vi "Write VI.vi"(8 "error in (no error)":errorcluster, 10 "VI Path (.vi)":path, 11 "Snippet":T1) -> (0 "error out":errorcluster)   [LabVIEW 2022 SP3, in "VI-Snippet.lvlib"]
doc: "Writes the embedded VI to disk."
uses:
  VI-Snippet.lvlib
  Snippet.ctl
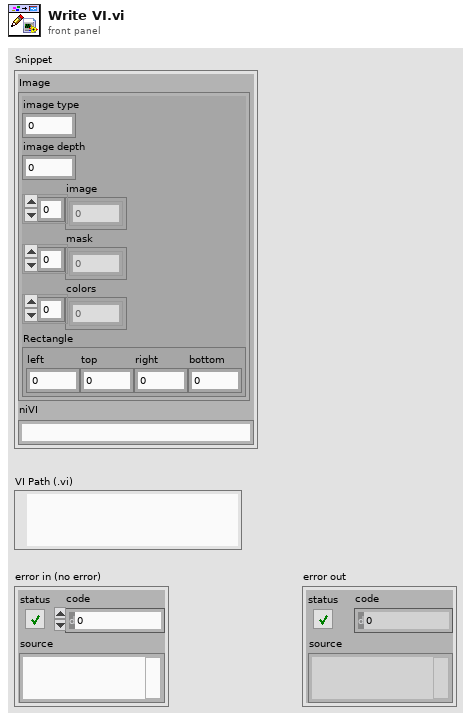
[diagram p1: front panel]
types:
  T1 = typedef "VI-Snippet.lvlib/Snippet.ctl" = cluster{"Image":cluster{"image type":i32, "image depth":i32, "image":u8[], "mask":u8[], "colors":u32[], "Rectangle":cluster{"left":i16, "top":i16, "right":i16, "bottom":i16}}, "niVI":string}
  T2 = enum16{"open", "replace", "create", "open or create", "replace or create", "replace or create with confirmation"}
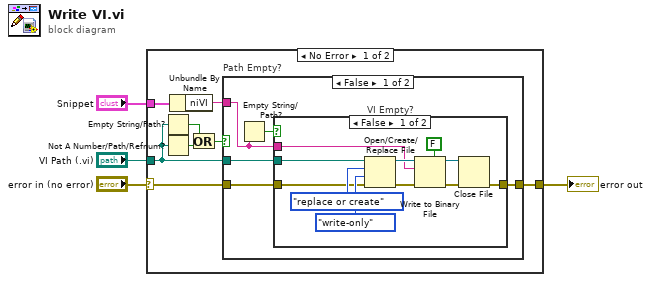
[diagram p0: block diagram]
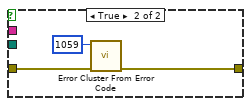
[diagram p2: hidden frame]
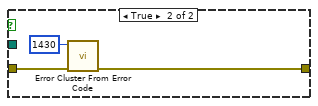
[diagram p3: hidden frame]
diagram:
  n1 = case shown="No Error" "error in (no error)" {
    selector: "error in (no error)" -> [w8 w35]
    tunnel: "Snippet" -> [w9 _]
    tunnel: [w12 w35] -> w3
    tunnel: "VI Path (.vi)" -> [w7 _]
    frame No Error {
      n2 = Empty String/Path?(string/path=w7) -> (empty?=w10:bool)
      n3 = Not A Number/Path/Refnum?(number/path/refnum=w7) -> (NaN/Path/Refnum?=w11:bool)
      n4 = Unbundle By Name(w9) -> ("niVI"=w6:string)
      n5 = Or(x=w10, y=w11) -> (x .or. y?=w5:bool)
      n6 = case "Path Empty?" shown="False" w5 {
        tunnel: [w17 w33] -> w12
        tunnel: w8 -> [w15 w32]
        tunnel: w7 -> [w16 _]
        tunnel: w6 -> [w14 _]
        frame False {
          n7 = Empty String/Path?(string/path=w14) -> (empty?=w13:bool)
          n8 = case "VI Empty?" shown="False" w13 {
            tunnel: [w28 w29] -> w17
            tunnel: w16 -> [w20 _]
            tunnel: w14 -> [w19 _]
            tunnel: w15 -> [w18 w30]
            frame False {
              n9 = Open/Create/Replace File(file path (use dialog)=w20, error in=w18, operation (0:open)=T2."replace or create", access (0:read/write)=enum16{"read/write", "read-only", "write-only"}."write-only") -> (refnum out=w23:refnum<file>, error out=w24:errorcluster)  [unwired: 2 in, 1 out]
              n10 = Write to Binary File(file (use dialog)=w23, data=w19, error in=w24, 5:FALSE ("prepend array or string size? (T)")) -> (refnum out=w26:refnum<file>, error out=w27:errorcluster)  [unwired: 2 in, 1 out]
              n11 = Close File(refnum=w26, error in=w27) -> (error out=w28:errorcluster)  [unwired: 1 out]
            }
            frame True {
              n12 = call <vilib>:"Error Cluster From Error Code.vi"("error in (no error)"=w30, "error code (0)"=1059 ("code")) -> ("error out"=w29:errorcluster)  [unwired: 7 in]
            }
          }
        }
        frame True {
          n13 = call <vilib>:"Error Cluster From Error Code.vi"("error in (no error)"=w32, "error code (0)"=1430 ("code")) -> ("error out"=w33:errorcluster)  [unwired: 7 in]
        }
      }
    }
    frame Error {
    }
  }
  "error out" <- w3
